vi "Get Components.vi"(8 "error in":errorcluster, 11 "board in":refnum<class "Board Design.lvclass">) -> (0 "error out":errorcluster, 2 "components":refnum<class "Component.lvclass">[](array[class]), 3 "board out":refnum<class "Board Design.lvclass">)   [LabVIEW 2023, in "Board Design.lvclass"]
doc: "Get an array of components for the board."
uses:
  Board Design.lvclass
  Component/Component.lvclass
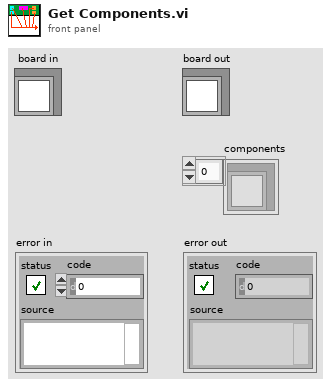
[diagram p1: front panel]
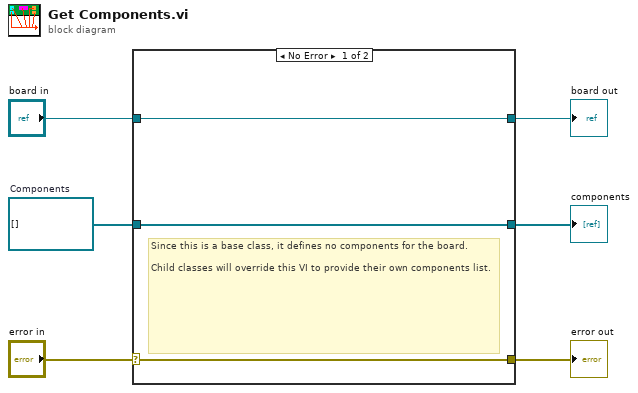
[diagram p0: block diagram]
diagram:
  w4 = refnum<class "Component.lvclass">[] []  # Components
  n1 = case shown="No Error" "error in" {
    selector: "error in" -> [w9 w10]
    tunnel: [w9 w10] -> w5
    tunnel: [w8 w11] -> w3
    tunnel: w4 -> [w8 w11]
    tunnel: "board in" -> [w7 w12]
    tunnel: [w7 w12] -> w1
    frame No Error {
      # "Since this is a base class, it defines no components for the board.\n\nChild classes will override this VI to provide their own components list."
    }
    frame Error {
    }
  }
  "error out" <- w5
  "board out" <- w1
  "components" <- w3
